vi "Get Channel Names and Default Values.vi"(8 "error in":errorcluster, 11 "module in":refnum<class "Module.lvclass">) -> (0 "error out":errorcluster, 1 "default values":dbl[](array[numeric]), 2 "names":string[](array[string]), 3 "module out":refnum<class "Module.lvclass">)   [LabVIEW 2017, in "Scan Engine Scripting.lvlib" / "Module.lvclass"]
uses:
  Module.lvclass
  Mode Classes/Mode/Mode.lvclass
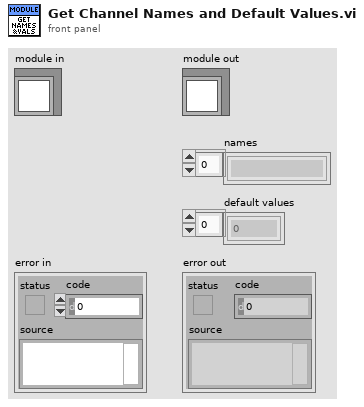
[diagram p1: front panel]
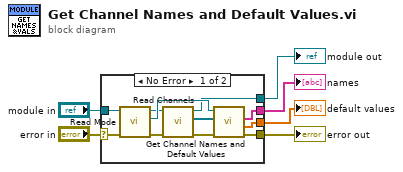
[diagram p0: block diagram]
diagram:
  n1 = case shown="No Error" "error in" {
    selector: "error in" -> [w10 w19]
    tunnel: [w9 w19] -> w5
    tunnel: [w14 w18] -> w3
    tunnel: "module in" -> [w17 w18]
    tunnel: [w8 _] -> w2
    tunnel: [w7 _] -> w1
    frame No Error {
      n2 = call-dynamic "Read Mode.vi"("error in"=w10, "module in"=w17) -> ("error out"=w11:errorcluster, "mode"=w16:refnum<class "Mode.lvclass">, "module out"=w15:refnum<class "Module.lvclass">)  [unwired: 7 in]
      n3 = call-dynamic "Read Channels.vi"("error in"=w11, "module in"=w15) -> ("error out"=w12:errorcluster, "channels"=w13:refnum<class "Channel.lvclass">[], "module out"=w14:refnum<class "Module.lvclass">)  [unwired: 7 in]
      n4 = call-dynamic "Get Channel Names and Default Values.vi"("error in"=w12, "channels"=w13, "mode in"=w16) -> ("error out"=w9:errorcluster, "default values"=w7:dbl[], "names"=w8:string[])  [unwired: 5 in, 1 out]
    }
    frame Error {
    }
  }
  "error out" <- w5
  "module out" <- w3
  "names" <- w2
  "default values" <- w1
